vi "GetRequest.vi"(10 "JSON string":string) -> (2 "request":T1)   [LabVIEW 2013]
panel:
  in  "request_cluster":T1
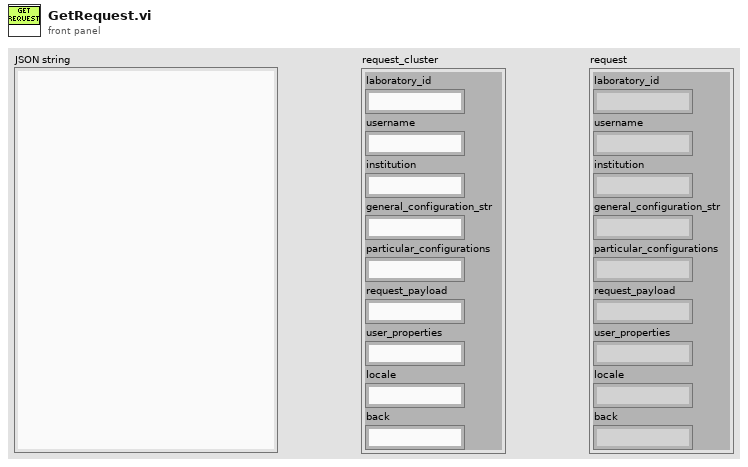
[diagram p1: front panel]
types:
  T1 = cluster{"laboratory_id":string, "username":string, "institution":string, "general_configuration_str":string, "particular_configurations":string, "request_payload":string, "user_properties":string, "locale":string, "back":string}
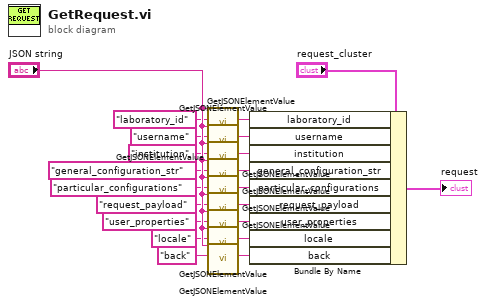
[diagram p0: block diagram]
diagram:
  n1 = call "GetJSONElementValue.vi"("JSON string"="JSON string", "JSON element name"="laboratory_id") -> ("JSON element value"=w12:string)  [unwired: 8 in, 1 out]
  n2 = call "GetJSONElementValue.vi"("JSON string"="JSON string", "JSON element name"="username") -> ("JSON element value"=w13:string)  [unwired: 8 in, 1 out]
  n3 = call "GetJSONElementValue.vi"("JSON string"="JSON string", "JSON element name"="institution") -> ("JSON element value"=w14:string)  [unwired: 8 in, 1 out]
  n4 = call "GetJSONElementValue.vi"("JSON string"="JSON string", "JSON element name"="general_configuration_str") -> ("JSON element value"=w15:string)  [unwired: 8 in, 1 out]
  n5 = call "GetJSONElementValue.vi"("JSON string"="JSON string", "JSON element name"="particular_configurations") -> ("JSON element value"=w16:string)  [unwired: 8 in, 1 out]
  n6 = call "GetJSONElementValue.vi"("JSON string"="JSON string", "JSON element name"="request_payload") -> ("JSON element value"=w17:string)  [unwired: 8 in, 1 out]
  n7 = call "GetJSONElementValue.vi"("JSON string"="JSON string", "JSON element name"="user_properties") -> ("JSON element value"=w18:string)  [unwired: 8 in, 1 out]
  n8 = call "GetJSONElementValue.vi"("JSON string"="JSON string", "JSON element name"="locale") -> ("JSON element value"=w19:string)  [unwired: 8 in, 1 out]
  n9 = call "GetJSONElementValue.vi"("JSON string"="JSON string", "JSON element name"="back") -> ("JSON element value"=w20:string)  [unwired: 8 in, 1 out]
  n10 = Bundle By Name(cluster="request_cluster", "laboratory_id"=w12, "username"=w13, "institution"=w14, "general_configuration_str"=w15, "particular_configurations"=w16, "request_payload"=w17, "user_properties"=w18, "locale"=w19, "back"=w20) -> (→"request":T1)
